vi "solar_misc Array Duplicates.vi"(10 "Array":string[](array[string])) -> (2 "Duplicates Removed":string[](array[string]), 5 "Unique Indexes":i32[](array[numeric]))   [LabVIEW 2018]
doc: "This removes duplicates in an array and returns their indexes."
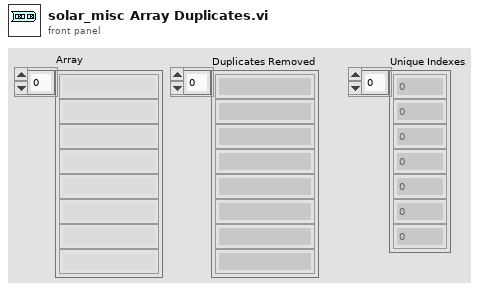
[diagram p1: front panel]
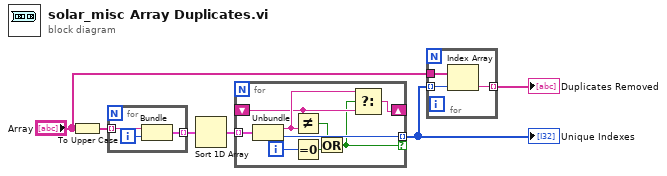
[diagram p0: block diagram]
diagram:
  n1 = To Upper Case(1:"Array") -> (0:w4:string[])
  n2 = for {
    tunnel: w4 -> [w9] mode=indexing
    tunnel: [w7] -> w5 mode=indexing
    i -> [w8]
    n3 = Bundle("String"=w9, w8) -> (w7:cluster{"String":string, i32})  [unwired: 1 in]
  }
  n4 = Sort 1D Array(array=w5) -> (sorted array=w6:cluster{"String":string, i32}[])
  n5 = for {
    tunnel: w6 -> [w18] mode=indexing
    tunnel: [w17] -> w3 mode=indexing if=w10
    shift-right: [w12] -> _
    shift-left: _ -> [w11]
    i -> [w16]
    n6 = Unbundle(w18) -> ("String"=w13:string, w17:i32)
    n7 = Not Equal?(x=w11, y=w13) -> (x != y?=w14:bool)
    n8 = Equal To 0?(x=w16) -> (x = 0?=w15:bool)
    n9 = Or(x=w14, y=w15) -> (x .or. y?=w10:bool)
    n10 = Select(t=w13, s=w10, f=w11) -> (s? t:f=w12:string)
  }
  "Unique Indexes" <- w3
  n11 = for {
    tunnel: w3 -> [w21] mode=indexing
    tunnel: "Array" -> [w20]
    tunnel: [w19] -> w1 mode=indexing
    n12 = Index Array(array=w20, index=w21) -> (element=w19:string)
  }
  "Duplicates Removed" <- w1
